vi "Serialize Data.vi"(8 "error in (no error)":errorcluster, 11 "Process Data":T1={"Sound Data"=[], "Sound Format"={"sample rate (S/s)"=22050.0, "number of channels"=2, "bits per sample"=16}}) -> (0 "error out":errorcluster, 3 "Flat Data out":string)   [LabVIEW 2020, in "Audio Data.lvlib"]
doc: "Version 0.1"
uses:
  <vilib>/ADAS Record/CustomDataTypes/Audio Data/Audio Data.lvlib
  69b4f655-d322-486f-8d65-ee31f7d8c6ef.vi
  <vilib>/ADAS Record/IODataPEF/CfgMgr/FlatFormat.ctl
  <vilib>/ADAS Record/CustomDataTypes/Audio Data/Process Data.ctl
  <vilib>/sound2/lvsound2.llb/Sound Data Format.ctl
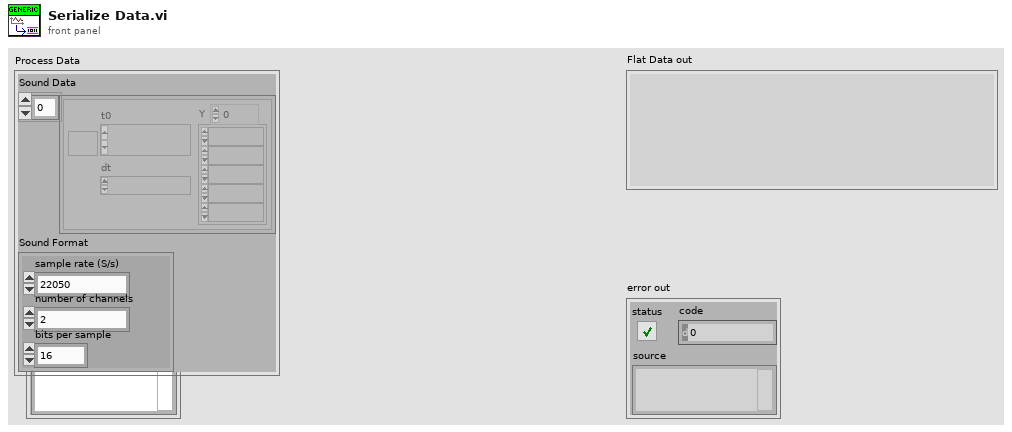
[diagram p1: front panel]
types:
  T1 = typedef "Audio Data.lvlib/Process Data.ctl" = cluster{"Sound Data":waveform(dbl)[], "Sound Format":T2}
  T2 = typedef "Sound Data Format.ctl" = cluster{"sample rate (S/s)":dbl, "number of channels":i32, "bits per sample":i32}
  T3 = typedef "FlatFormat.ctl" = enum32{"Auto", "PEF", "GFB (Apache)", "GFB", "JSON", "Readable JSON", "LV String", "Reserved", "LV Native"}
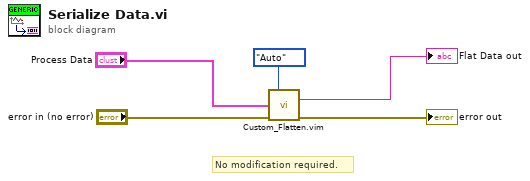
[diagram p0: block diagram]
diagram:
  # "No modification required."
  n1 = call "Custom_Flatten.vim"("Flat Format"=FlatFormat."Auto", "Data"="Process Data", "error in (no error)"="error in (no error)") -> ("Flat Data"=→"Flat Data out":string, "Error (out)"=→"error out":errorcluster)  [unwired: 10 in, 1 out]
